vi "Load Files to Ring Control.vi"(8 "Error in":errorcluster, 11 "Ring in":refnum<vi>) -> (0 "error out":errorcluster, 2 "Path to files":path, 3 "Ring out":refnum<vi>)   [LabVIEW 2018]
doc: "this VI takes the reference to a ring control and loads the array of options based on the files available at the auto/populating folder"
uses:
  <vilib>/Utility/sysdir.llb/System Directory Type.ctl
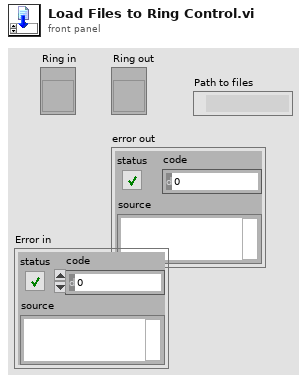
[diagram p1: front panel]
types:
  T1 = typedef "System Directory Type.ctl" = i32
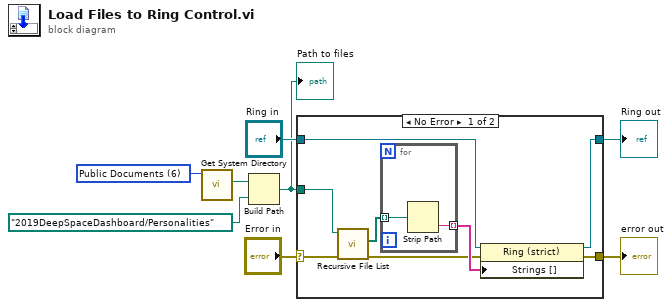
[diagram p0: block diagram]
diagram:
  w1 = T1 6 items=["User Home"=0, "User Desktop"=1, "User Documents"=2, "User Application Data"=3, "User Preferences"=4, "User Temporary"=5, "Public Documents"=6, "Public Application Data"=7, "Public Preferences"=8, "Public Cache"=13, "System Core Libraries"=9, "System Installed Libraries"=10, "Application Files"=11, "Boot Volume Root"=12] ("system directory type")
  n1 = call <vilib>:"Get System Directory.vi"("system directory type"=w1) -> ("system directory"=w2:path)  [unwired: 10 in]
  n2 = Build Path(base path=w2, name or relative path=path "2019DeepSpaceDashboard/Personalities" ("appended path")) -> (appended path=w4:path)
  "Path to files" <- w4
  n3 = case shown="No Error" "Error in" {
    selector: "Error in" -> [w9 w20]
    tunnel: [w14 w20] -> w8
    tunnel: [w12 w19] -> w7
    tunnel: "Ring in" -> [w11 w19]
    tunnel: w4 -> [w10 _]
    frame No Error {
      n4 = call <vilib>:"Recursive File List.vi"("error in (no error)"=w9, "Folder Path"=w10) -> ("error out"=w13:errorcluster, "All Files in Dir"=w15:path[])  [unwired: 5 in, 3 out]
      n5 = for {
        tunnel: [w17] -> w16 mode=indexing
        tunnel: w15 -> [w18] mode=indexing
        n6 = Strip Path(path=w18) -> (name=w17:string)  [unwired: 1 out]
      }
      n7 = property class="Ring (strict)"(reference=w11, error in=w13, "Strings []"=w16) -> (reference out=w12:refnum<vi>, error out=w14:errorcluster)
    }
    frame Error {
    }
  }
  "error out" <- w8
  "Ring out" <- w7
